vi "Intake Logic.vi"(1 "Operator Intake In":T3) -> (0 "Operator Intake Out":T3)   [LabVIEW 2013]
uses:
  <vilib>/Rock Robotics/WPI/Relay/WPI_RelayValue.ctl
  <vilib>/Rock Robotics/WPI/Solenoid/WPI_SolenoidValue.ctl
  Cannon/Cannon Global.vi
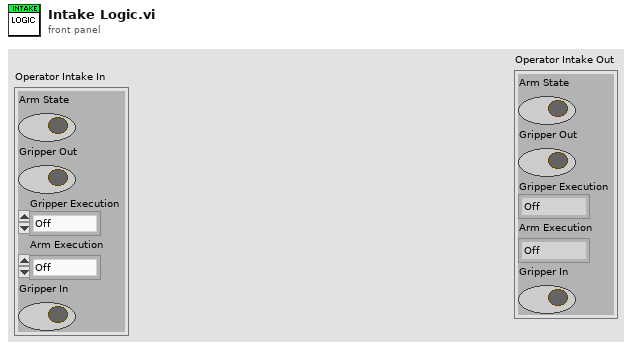
[diagram p1: front panel]
types:
  T1 = typedef "WPI_RelayValue.ctl" = enum16{"Off", "On", "Forward", "Reverse"}
  T2 = typedef "WPI_SolenoidValue.ctl" = enum16{"Off", "On", "Forward", "Reverse"}
  T3 = cluster{"Arm State":bool, "Gripper Out":bool, "Gripper Execution":T1, "Arm Execution":T2, "Gripper In":bool}
  T4 = cluster{"Angle":dbl, "Clutch MS":bool, "Ball MS":bool, "Clutch ":T1, "LeFireatwill":bool, "Arm":bool, "Armed":bool, "Fire!":bool, "Bottom MS":bool, "Motor VBus":dbl}
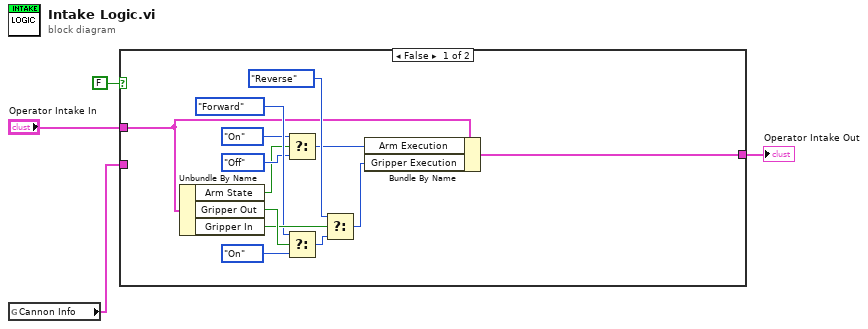
[diagram p0: block diagram]
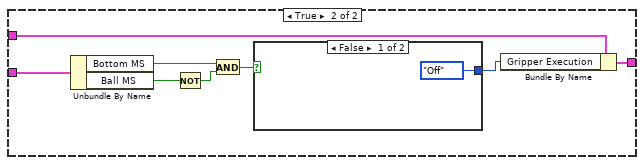
[diagram p2: hidden frame]
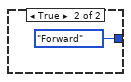
[diagram p3: hidden frame]
diagram:
  n1 = global read "Cannon Global.vi" "Cannon Info"() -> (w1:T4)
  n2 = case shown="False" FALSE {
    tunnel: [w7 w20] -> w4
    tunnel: "Operator Intake In" -> [w8 w19]
    tunnel: w1 -> [_ w18]
    frame False {
      n3 = Unbundle By Name(w8) -> ("Arm State"=w5:bool, "Gripper Out"=w17:bool, "Gripper In"=w16:bool)
      n4 = Select(t=WPI_RelayValue."On" ("Gripper Execution"), s=w5, f=WPI_RelayValue."Off" ("Gripper Execution")) -> (s? t:f=w6:T1)
      n5 = Select(t=WPI_RelayValue."Forward" ("Gripper Execution"), s=w17, f=WPI_RelayValue."On" ("Gripper Execution")) -> (s? t:f=w14:T1)
      n6 = Select(t=WPI_RelayValue."Reverse" ("Gripper Execution"), s=w16, f=w14) -> (s? t:f=w15:T1)
      n7 = Bundle By Name(cluster=w8, "Arm Execution"=w6, "Gripper Execution"=w15) -> (w7:T3)
    }
    frame True {
      n8 = Unbundle By Name(w18) -> ("Bottom MS"=w25:bool, "Ball MS"=w23:bool)
      n9 = Not(x=w23) -> (.not. x?=w24:bool)
      n10 = And(x=w25, y=w24) -> (x .and. y?=w22:bool)
      n11 = case shown="False" w22 {
        tunnel: [WPI_RelayValue."Off" ("Gripper Execution") WPI_RelayValue."Forward" ("Gripper Execution")] -> w21
        frame False {
        }
        frame True {
        }
      }
      n12 = Bundle By Name(cluster=w19, "Gripper Execution"=w21) -> (w20:T3)
    }
  }
  "Operator Intake Out" <- w4
